vi "624 Safe Image Get Image.vi"(6 "Video Mode":i32, 8 "error in":errorcluster, 9 "Operation":T3(ring), 10 "Image In":T1, 11 "Session In":T2) -> (0 "error out":errorcluster, 1 "Image Data String":string, 2 "Image Out":T1, 3 "Session Out":T2)   [LabVIEW 2014]
uses:
  <vilib>/userdefined/High Color/IMAQdx.ctl
  <vilib>/vision/Image Controls.llb/IMAQ Image.ctl
  <vilib>/vision/driver/IMAQdx.llb/IMAQdx Buffer Number Mode.ctl
  <resource>/objmgr/imaqdx.rc
  <vilib>/vision/driver/NI_Vision_Acquisition_Software.lvlib
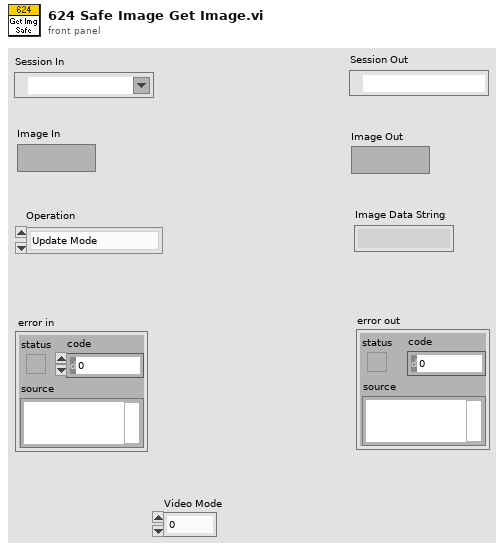
[diagram p1: front panel]
types:
  T1 = typedef "IMAQ Image.ctl" = refnum<image>
  T2 = typedef "IMAQdx.ctl" = refnum<k21>
  T3 = enum16{"Update Mode", "Get Image", "Get Image Data"}
  T4 = typedef "NI_Vision_Acquisition_Software.lvlib/IMAQdx Buffer Number Mode.ctl" = enum32{"Next", "Last", "Buffer Number"}
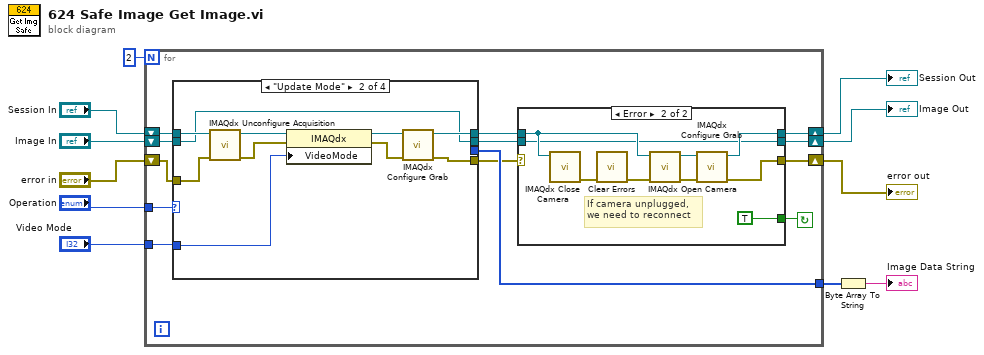
[diagram p0: block diagram]
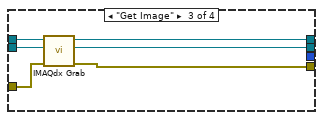
[diagram p4: hidden frame]
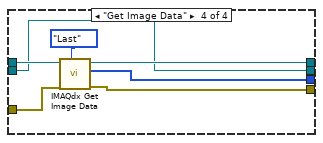
[diagram p5: hidden frame]
diagram:
  n1 = for {
    N: 2 -> [_]
    tunnel: "Operation" -> [w24]
    tunnel: "Video Mode" -> [w23]
    tunnel: [w19] -> w6
    shift-right: [w13] -> w2
    shift-left: "Session In" -> [w22]
    shift-right: [w15] -> w3
    shift-left: "Image In" -> [w21]
    shift-right: [w17] -> w4
    shift-left: "error in" -> [w20]
    stop <- w12 continue-if-true
    n2 = case shown="\"Update Mode\"" w24 {
      tunnel: w22 -> [w39 w49 w55 w58]
      tunnel: [w39 w46 w52 w60] -> w14
      tunnel: [w38 w44 w50 w59] -> w18
      tunnel: w23 -> [_ w42 _ _]
      tunnel: w21 -> [w37 w40 w54 w56]
      tunnel: [w37 w40 w51 w56] -> w16
      tunnel: [_ _ _ w61] -> w19
      tunnel: w20 -> [w38 w41 w53 w57]
      frame Default {
      }
      frame "Update Mode" {
        n3 = call <vilib>:"IMAQdx Unconfigure Acquisition.vi"("error in"=w41, "Session In"=w49) -> ("error out"=w43:errorcluster, "Session Out"=w48:T2)  [unwired: 8 in]
        n4 = property class="IMAQdx"(reference=w48, error in=w43, "VideoMode"=w42) -> (reference out=w47:T2, error out=w45:errorcluster)
        n5 = call <vilib>:"IMAQdx Configure Grab.vi"("error in"=w45, "Session In"=w47) -> ("error out"=w44:errorcluster, "Session Out"=w46:T2)  [unwired: 8 in]
      }
      frame "Get Image" {
        n6 = call <vilib>:"IMAQdx Grab.vi"("error in"=w53, "Image In"=w54, "Session In"=w55) -> ("error out"=w50:errorcluster, "Image Out"=w51:T1, "Session Out"=w52:T2)  [unwired: 5 in, 1 out]
      }
      frame "Get Image Data" {
        n7 = call <vilib>:"IMAQdx Get Image Data.vi"("Buffer Number Mode (Next)"=IMAQdx_Buffer_Number_Mode."Last", "error in"=w57, "Session In"=w58) -> ("error out"=w59:errorcluster, "Image Data Array"=w61:u8[], "Session Out"=w60:T2)  [unwired: 5 in, 1 out]
      }
    }
    n8 = case shown="Error" w18 {
      selector: w18 -> [w27 _]
      tunnel: [w27 w29] -> w17
      tunnel: w16 -> [w26 w30]
      tunnel: [w26 w30] -> w15
      tunnel: w14 -> [w25 w34]
      tunnel: [w25 w31] -> w13
      tunnel: [_ TRUE] -> w12
      frame No Error {
      }
      frame Error {
        # "If camera unplugged,\nwe need to reconnect"
        n9 = call <vilib>:"IMAQdx Close Camera.vi"("Session In"=w34) -> ("error out"=w33:errorcluster)  [unwired: 10 in]
        n10 = call <vilib>:"Clear Errors.vi"("error in (no error)"=w33) -> ("error out"=w32:errorcluster)  [unwired: 5 in, 1 out]
        n11 = call <vilib>:"IMAQdx Open Camera.vi"("error in"=w32, "Session In"=w34) -> ("error out"=w36:errorcluster, "Session Out"=w35:T2)  [unwired: 8 in]
        n12 = call <vilib>:"IMAQdx Configure Grab.vi"("error in"=w36, "Session In"=w35) -> ("error out"=w29:errorcluster, "Session Out"=w31:T2)  [unwired: 8 in]
      }
    }
  }
  "Session Out" <- w2
  "Image Out" <- w3
  "error out" <- w4
  n13 = Byte Array To String(unsigned byte array=w6) -> (string=→"Image Data String":string)
